vi "Write DevID.vi"(8 "error in (no error)":errorcluster, 10 "DevID":string, 11 "Update TEC PID in":refnum<class "Update TEC PID.lvclass">) -> (0 "error out":errorcluster, 3 "Update TEC PID out":refnum<class "Update TEC PID.lvclass">)   [LabVIEW 2014, in "Controller.lvlib" / "Update TEC PID.lvclass"]
uses:
  Update TEC PID.lvclass
  Update TEC PID.lvclass/Update TEC PID.ctl
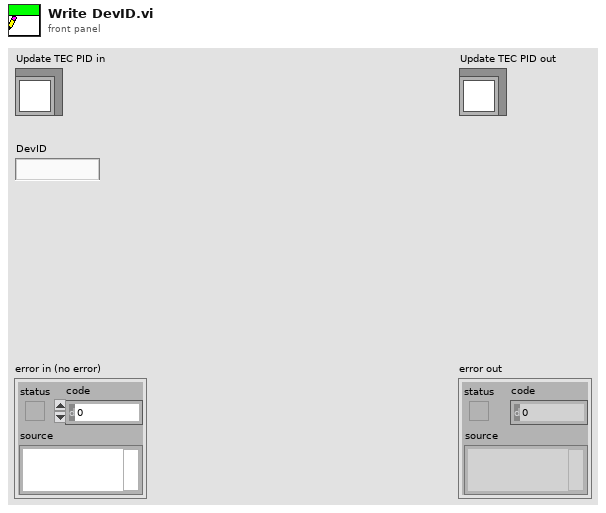
[diagram p1: front panel]
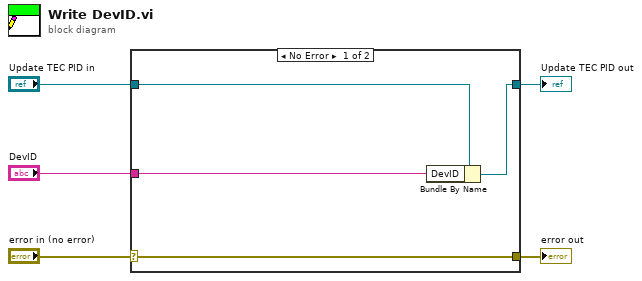
[diagram p0: block diagram]
diagram:
  n1 = case shown="No Error" "error in (no error)" {
    selector: "error in (no error)" -> [w9 w10]
    tunnel: [w9 w10] -> w4
    tunnel: [w7 w11] -> w2
    tunnel: "Update TEC PID in" -> [w8 w11]
    tunnel: "DevID" -> [w6 _]
    frame No Error {
      n2 = Bundle By Name(cluster=w8, "DevID"=w6) -> (w7:refnum<class "Update TEC PID.lvclass">)
    }
    frame Error {
    }
  }
  "error out" <- w4
  "Update TEC PID out" <- w2
